vi "DMM Fringe v01.vi"() -> ()   [LabVIEW 2010]
panel:
  out "max value":dbl
  out "x .or. y?":bool
  out "Midpoint":dbl
  out "min value":dbl
  out "Fringe Size (Vpp)":dbl
  in  "stop":bool
  out "Waveform Chart":dbl(graph)
  in  "milliseconds to wait":u32=20
  out "# of points taken":i32
  out "Value":dbl
  out "Reading (string)":string
  out "substring (Units)":string
  out "error out":errorcluster
  out "read buffer":string
  out "return count":u32
  in  "byte count":u32=5000000
  in  "VISA resource name":refnum<visa-resource-name>="GPIB0::25::INSTR"
  in  "write buffer":string="G0"
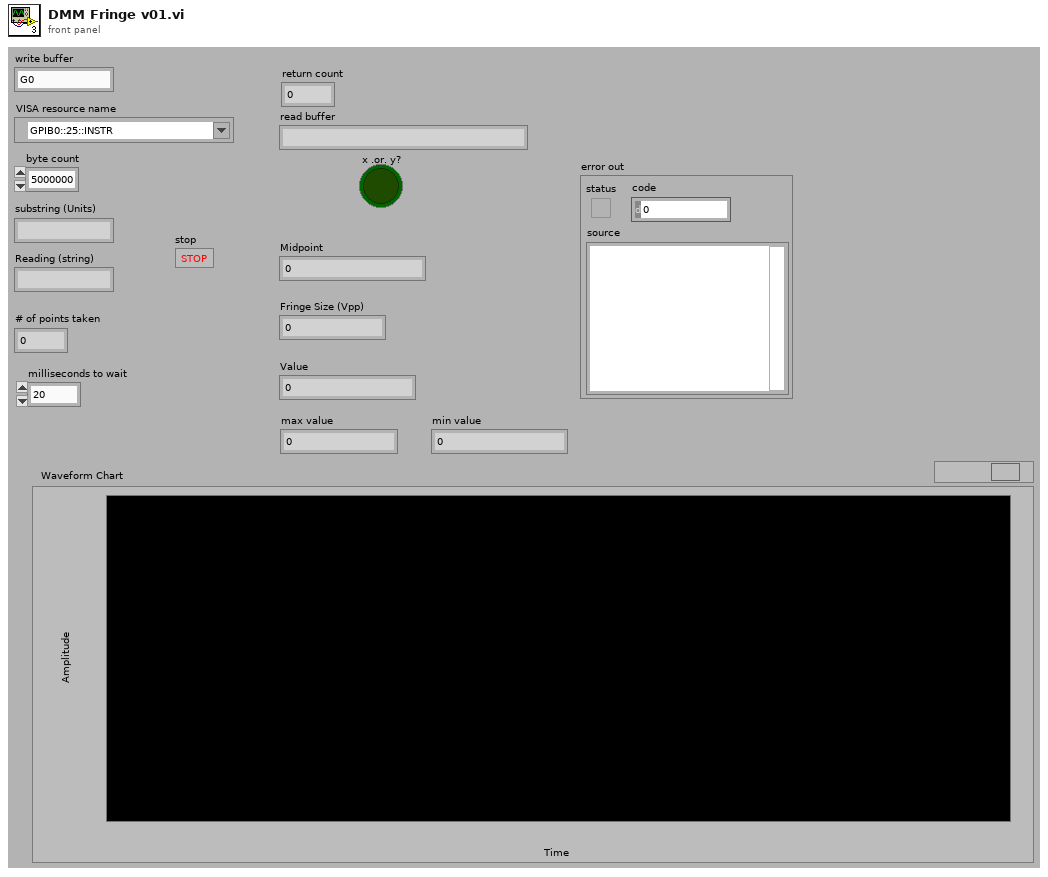
[diagram p1: front panel]
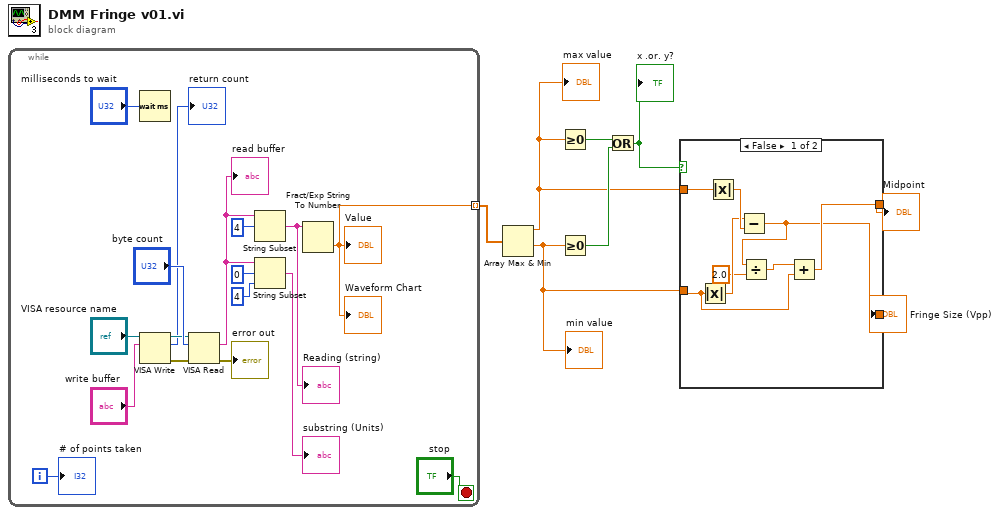
[diagram p0: block diagram]
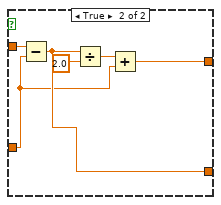
[diagram p2: hidden frame]
diagram:
  n1 = while {
    tunnel: [w9] -> w8 mode=indexing
    i -> [w12]
    stop <- "stop" stop-if-true
    n2 = Wait (ms)(milliseconds to wait="milliseconds to wait") -> ()  [unwired: 1 out]
    n3 = VISA Write(VISA resource name="VISA resource name", write buffer="write buffer") -> (VISA resource name out=w22:refnum<visa-resource-name>, return count=→"return count":u32, error out=w20:errorcluster)  [unwired: 1 in]
    n4 = VISA Read(VISA resource name=w22, byte count="byte count", error in (no error)=w20) -> (read buffer=w15:string, error out=→"error out":errorcluster)  [unwired: 2 out]
    "read buffer" <- w15
    n5 = String Subset(string=w15, offset (0)=4) -> (substring=w13:string)  [unwired: 1 in]
    "Reading (string)" <- w13
    n6 = String Subset(string=w15, offset (0)=0, length (rest)=4 ("length (rest)")) -> (substring=→"substring (Units)":string)
    n7 = Fract/Exp String To Number(string=w13) -> (number=w9:dbl)  [unwired: 3 in, 1 out]
    "Value" <- w9
    "Waveform Chart" <- w9
    "# of points taken" <- w12
  }
  n8 = Array Max & Min(array=w8) -> (max value=w3:dbl, min value=w4:dbl)  [unwired: 2 out]
  "min value" <- w4
  "max value" <- w3
  n9 = Greater Or Equal To 0?(x=w3) -> (x >= 0?=w6:bool)
  n10 = Greater Or Equal To 0?(x=w4) -> (x >= 0?=w5:bool)
  n11 = Or(x=w6, y=w5) -> (x .or. y?=w7:bool)
  "x .or. y?" <- w7
  n12 = case shown="False" w7 {
    tunnel: w4 -> [w29 w34]
    tunnel: w3 -> [w33 w37]
    tunnel: [w27 w36] -> w2
    tunnel: [w28 w35] -> w1
    frame False {
      n13 = Absolute Value(x=w29) -> (abs(x)=w31:dbl)
      n14 = Absolute Value(x=w33) -> (abs(x)=w32:dbl)
      n15 = Subtract(x=w31, y=w32) -> (x-y=w27:dbl)
      n16 = Divide(x=w27, y=2.0) -> (x/y=w30:dbl)
      n17 = Add(x=w30, y=w29) -> (x+y=w28:dbl)
    }
    frame True {
      n18 = Subtract(x=w37, y=w34) -> (x-y=w36:dbl)
      n19 = Divide(x=w36, y=2.0) -> (x/y=w39:dbl)
      n20 = Add(x=w39, y=w34) -> (x+y=w35:dbl)
    }
  }
  "Midpoint" <- w1
  "Fringe Size (Vpp)" <- w2
